vi "Read Poll List.vi"(8 "error in (no error)":errorcluster, 11 "MB PLC Client in":refnum<class "MB PLC Client.lvclass">) -> (0 "error out":errorcluster, 2 "Poll List":T1[](array[typedef]), 3 "MB PLC Client out":refnum<class "MB PLC Client.lvclass">)   [LabVIEW 2018, in "MB PLC Client.lvlib" / "MB PLC Client.lvclass"]
uses:
  MB PLC Client.lvclass
  Types/MB Ref Range_Cluster.ctl
  MB PLC Client.lvclass/MB PLC Client.ctl
  MB PLC Client.lvlib
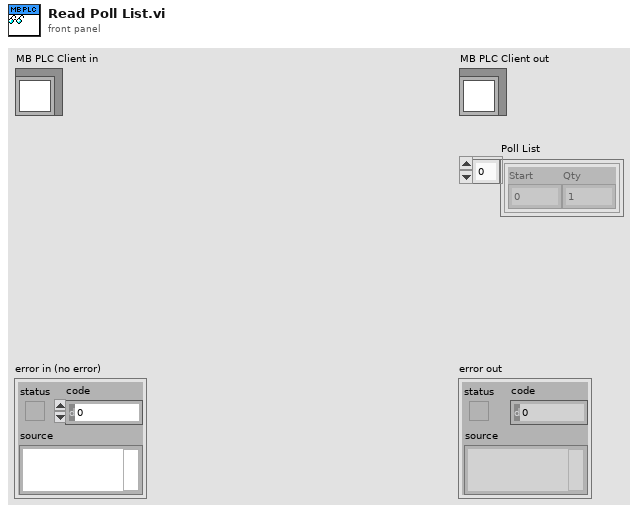
[diagram p1: front panel]
types:
  T1 = typedef "MB PLC Client.lvlib/MB Ref Range_Cluster.ctl" = cluster{"Start":u32, "Qty":u16}
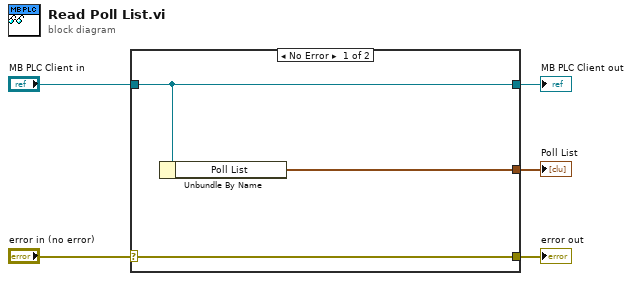
[diagram p0: block diagram]
diagram:
  n1 = case shown="No Error" "error in (no error)" {
    selector: "error in (no error)" -> [w8 w9]
    tunnel: [w8 w9] -> w4
    tunnel: [w7 w10] -> w2
    tunnel: "MB PLC Client in" -> [w7 w10]
    tunnel: [w6 _] -> w1
    frame No Error {
      n2 = Unbundle By Name(w7) -> ("Poll List"=w6:T1[])
    }
    frame Error {
    }
  }
  "error out" <- w4
  "MB PLC Client out" <- w2
  "Poll List" <- w1
